vi "OnDataChange.vi"(0 "GRMActor in":refnum<class "Displayer.lvclass">, 1 "DataExchange":T1, 3 "error in (no error)":errorcluster) -> (7 "GRMActor out":refnum<class "Displayer.lvclass">, 10 "error out":errorcluster)   [LabVIEW 2020, in "Displayer.lvlib" / "Displayer.lvclass"]
uses:
  Displayer.lvclass
  Model/Hardware Abstraction Layer/Component/Device/Device/DataExchange.ctl
  Model/Hardware Abstraction Layer/Component/GenericActor/GenericActor/GenericActor.lvclass
  Interface/DataListener/DataListener.lvclass
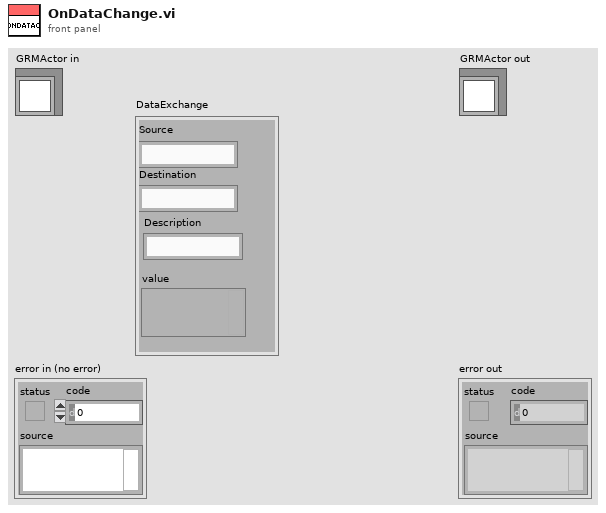
[diagram p1: front panel]
types:
  T1 = typedef "DataListener.lvclass/DataExchange.ctl" = cluster{"Source":string, "Destination":string, "Description":string, "value":variant}
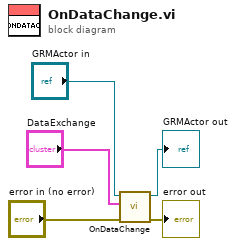
[diagram p0: block diagram]
diagram:
  n1 = call-parent "OnDataChange.vi"("GRMActor in"="GRMActor in", "DataExchange"="DataExchange", "error in (no error)"="error in (no error)") -> ("GRMActor out"=→"GRMActor out":refnum<class "Displayer.lvclass">, "error out"=→"error out":errorcluster)  [unwired: 6 in]
